vi "MEASURE_hysteresis_multiple_SHG gate_pmt.vi"() -> ()   [LabVIEW 2020]
uses:
  <vilib>/DAQmx/read.llb/DAQmx Read.vi
  <vilib>/DAQmx/read.llb/DAQmx Read (Counter U32 1Chan 1Samp).vi
  <vilib>/DAQmx/create/channels.llb/DAQmx Create Channel (CI-Count Edges).vi
  <vilib>/DAQmx/miscellaneous.llb/DAQmx Fill In Error Info.vi
  <vilib>/Utility/file.llb/Write To Spreadsheet File (DBL).vi
  <instrlib>/Stanford Research 830/Stanford Research 830.lvlib
  <instrlib>/Keithley 2450/Keithley 2450.lvlib
  <resource>/objmgr/daqmx.rc
panel:
  out "XY Graph 2":cluster{dbl[], dbl[]}(graph)
  in  "accumulation":i32=20
  in  "Interval (ms)":i32=20
  out "error out":errorcluster
  in  "Counter Channel":tag="/Dev1/PFI0"
  in  "error in":errorcluster
  out "loop run":i32
  in  "loop #":i32
  in  "Save data or not":bool=TRUE
  in  "path (folder + filename)":string="D:\\Kedar\\MoS2\\jw7_DJ_bulk_111213\\VvsHtr\\VvsHtr_300K"
  in  "Clear Plot":bool
  out "XY Graph":cluster{dbl[], dbl[]}(graph)
  out "LOCKIN Measurement":dbl
  in  "Parameter (1: X)":u16(ring)=1 items=["X"=1, "Y"=2, "R"=3, "Theta"=4, "Channel 1"=5, "Channel 2"=6, "Aux In 1"=7, "Aux In 2"=8, "Aux In 3"=9, "Aux In 4"=10]
  out "gate voltage":dbl format="%#_13g"
  out "gate leaking":string="defbuffer1"
  in  "GATE STEP(mv)":i32
  in  "GATE Low Value (default 0)":dbl=1.0
  in  "GATE High Value":dbl=1.0
  in  "Function (0: Volts) 2":u16(ring) items=["Volts", "Current", "Resistance"]
  in  "Source Compaliance":dbl=1e-06
  in  "V address":refnum<visa-resource-name>="GPIB0::24::INSTR"
  in  "SD stabilization(S) 2":dbl format="%#_13g"
  in  "Sine Output Amplitude (1 V) 2":dbl=1.0
  in  "GATE / SD stablization 3":dbl format="%#_13g"
  in  "frequency":dbl format="%#_13g"
  in  "Input Connection (0: Single-Ended Voltage)":u16(ring) items=["Single-Ended Voltage", "Differential Voltage", "1 MOhm Current Gain", "100 MOhm Current Gain"]
  in  "LOCKIN address":refnum<visa-resource-name>="GPIB0::24::INSTR"
  # "Lock-in"
  # "Gate Setting"
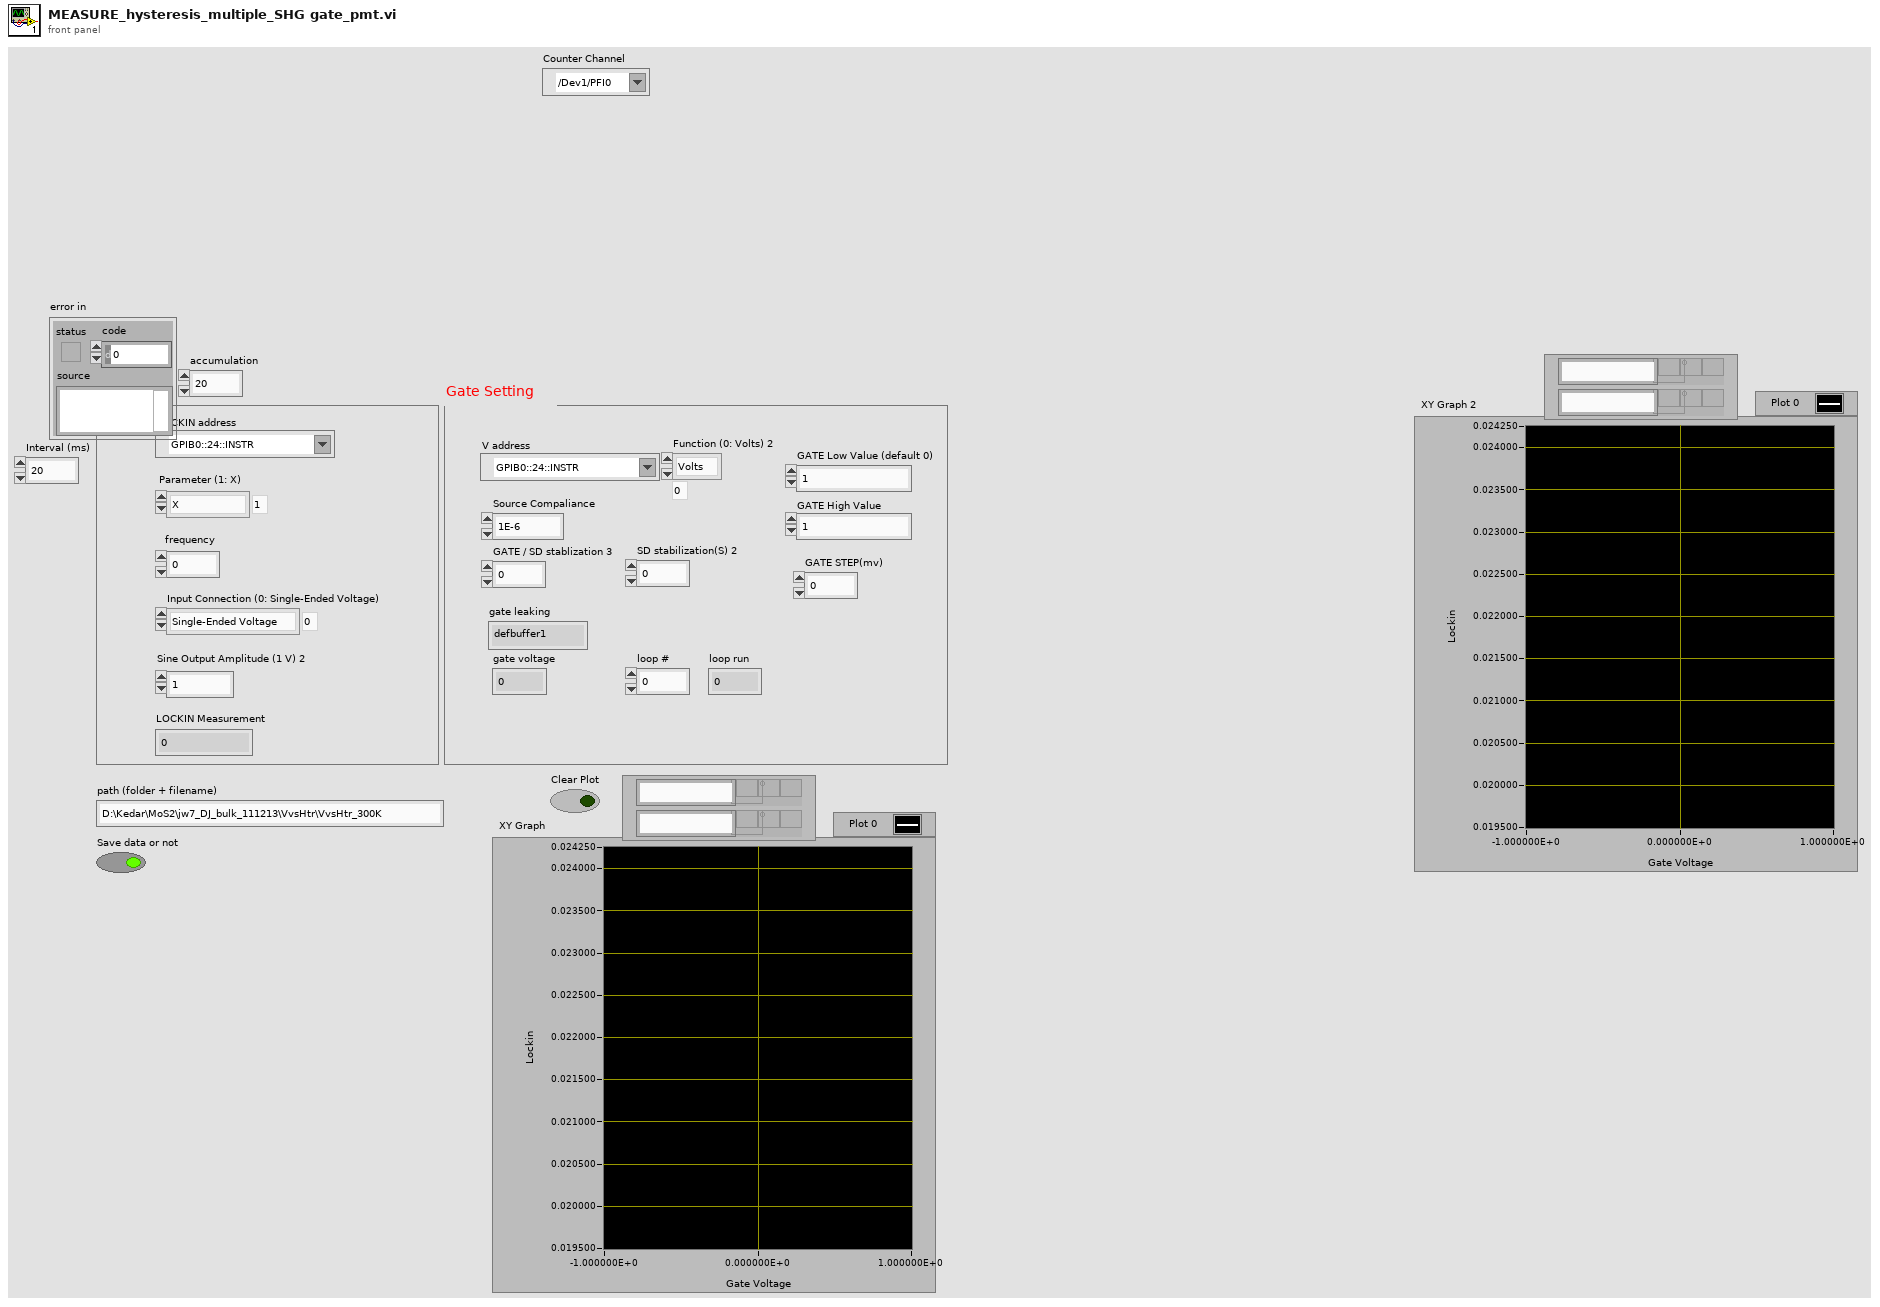
[diagram p1: front panel]
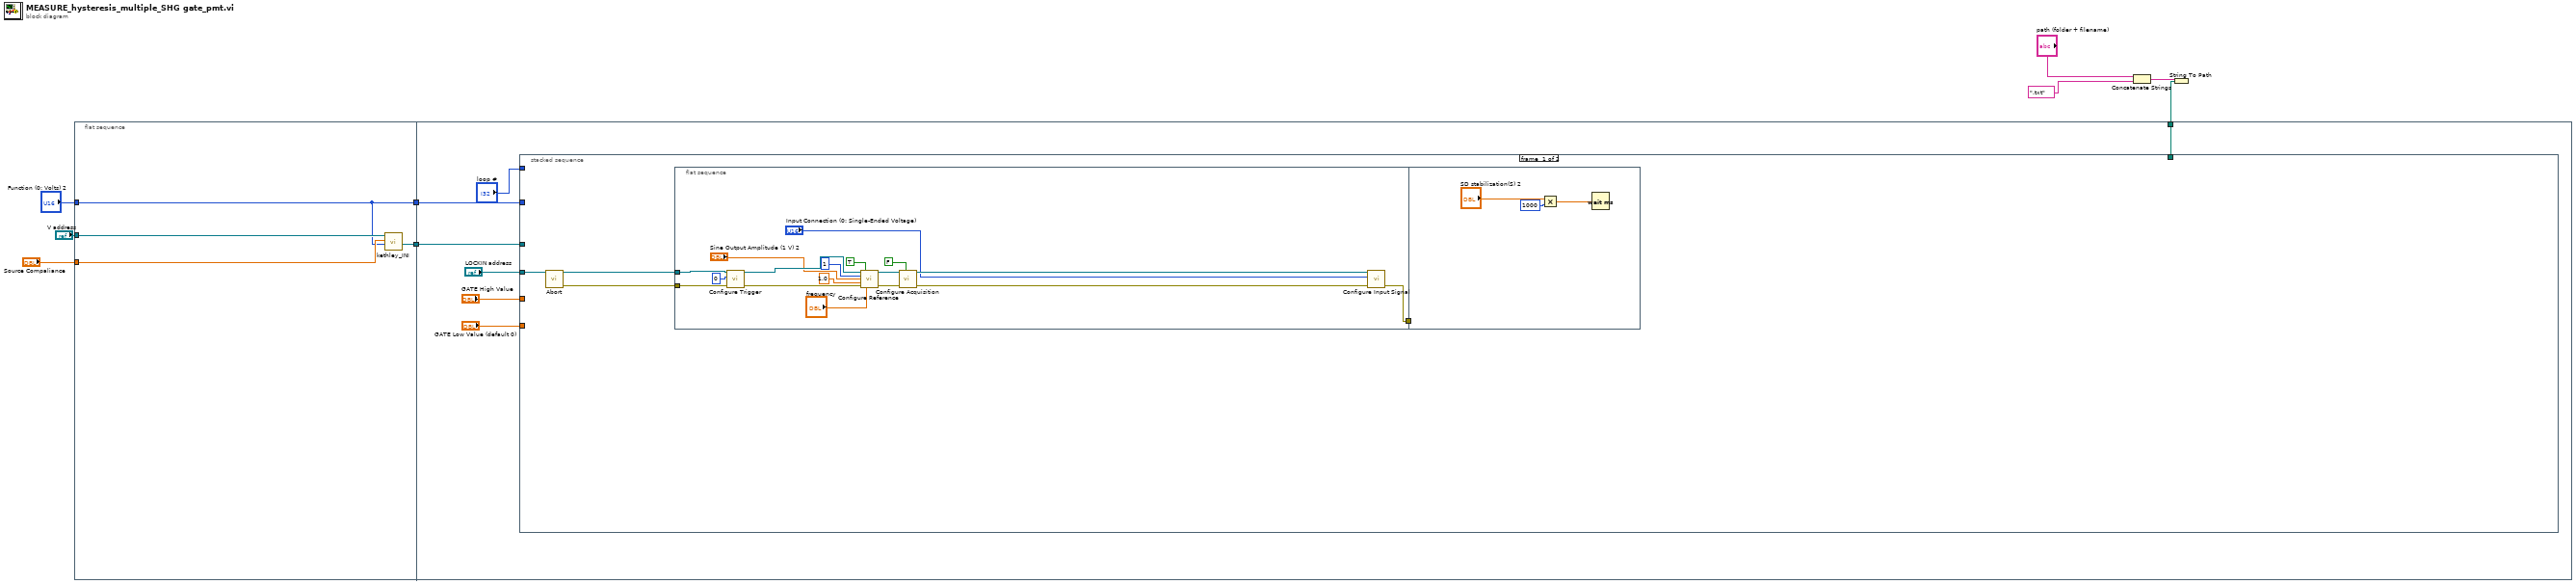
[diagram p0: block diagram]
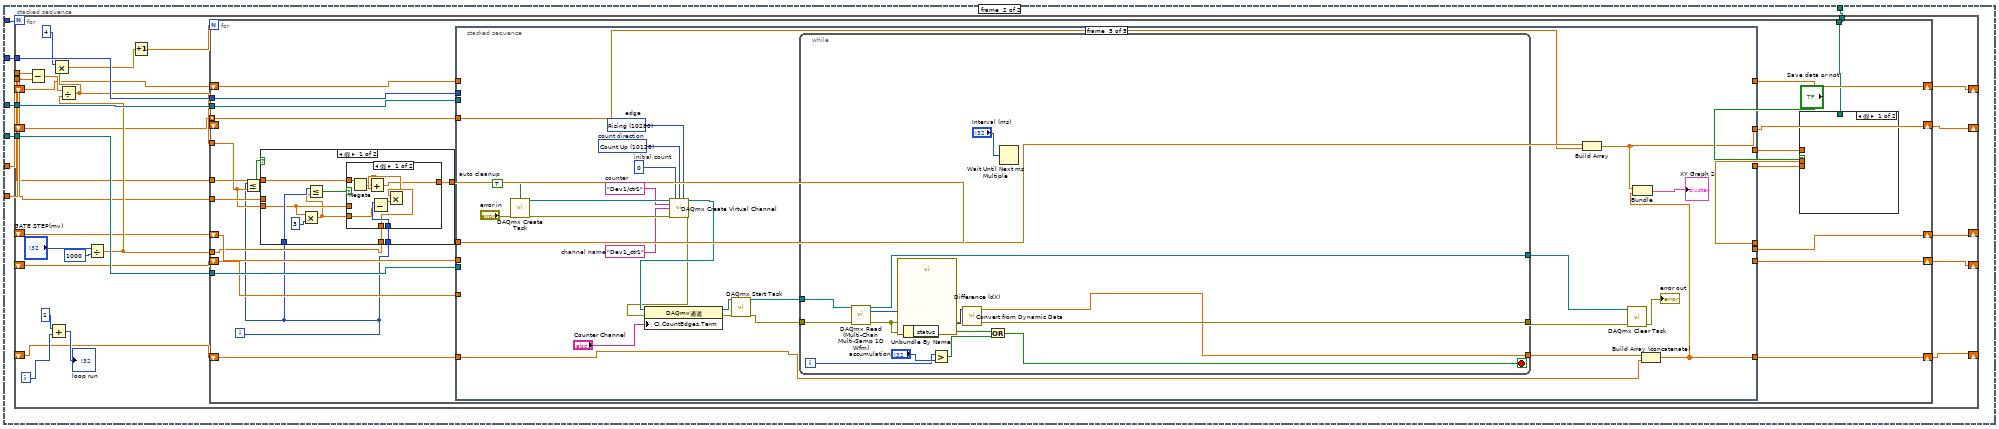
[diagram p2: hidden frame]
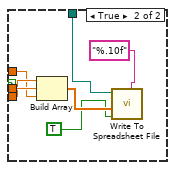
[diagram p3: hidden frame]
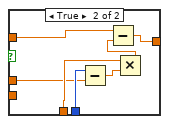
[diagram p4: hidden frame]
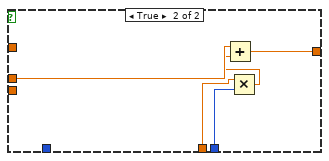
[diagram p5: hidden frame]
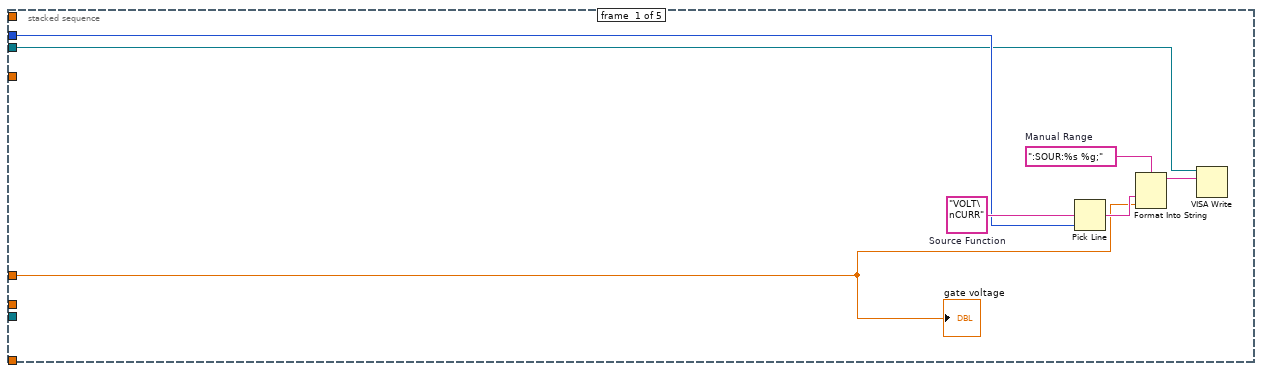
[diagram p6: hidden frame]
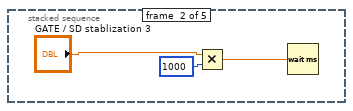
[diagram p7: hidden frame]
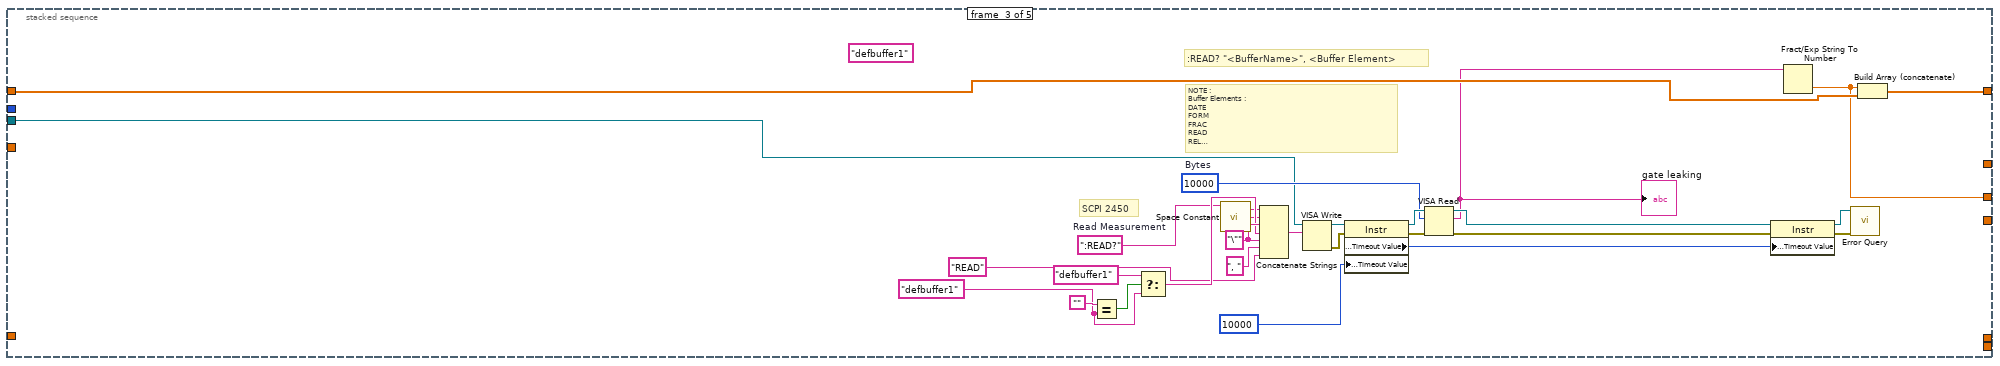
[diagram p8: hidden frame]
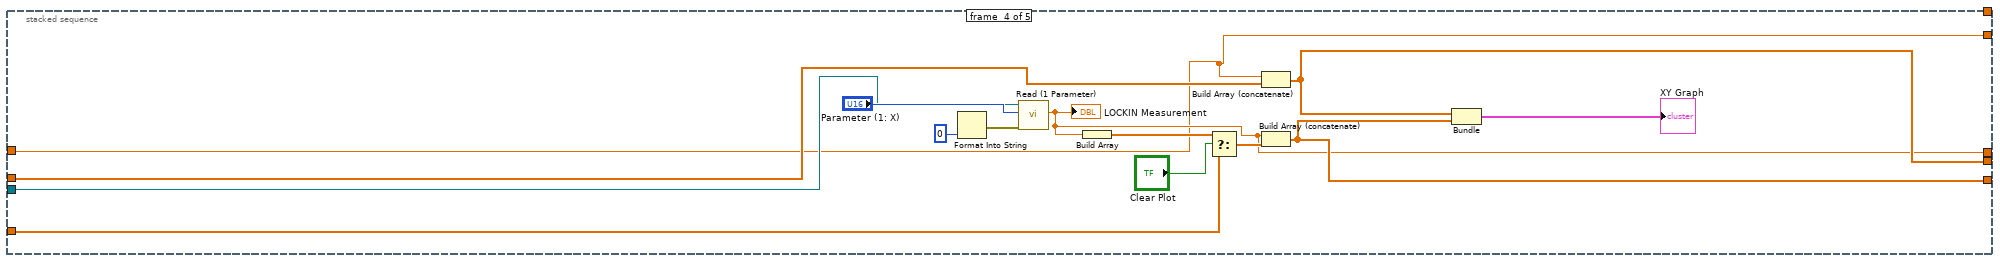
[diagram p9: hidden frame]
diagram:
  n1 = flat-sequence {
    tunnel: "V address" -> [w13]
    tunnel: "Source Compaliance" -> [w12]
    tunnel: "Function (0: Volts) 2" -> [w10]
    tunnel: [w11] -> w6
    tunnel: [w10] -> w5
    tunnel: w6 -> [w19]
    tunnel: w5 -> [w18]
    tunnel: w1 -> [w15]
    frame #0 {
      n2 = call "kethley_INI.vi"("Function (0: Volts) in"=w10, "Source Compaliance"=w12, "VISA Refnum in"=w13) -> ("VISA resource name out"=w11:refnum<visa-resource-name>)  [unwired: 8 in]
    }
    frame #1 {
      n3 = stacked-sequence {
        tunnel: "LOCKIN address" -> [w23 w49]
        tunnel: w19 -> [_ w50]
        tunnel: w18 -> [_ w51]
        tunnel: "GATE High Value" -> [_ w47]
        tunnel: "GATE Low Value (default 0)" -> [_ w48]
        tunnel: w15 -> [_ w46]
        tunnel: "loop #" -> [_ w45]
        frame #0 {
          n4 = call <instrlib>:"Abort.vi"("VISA resource name"=w23) -> ("error out"=w21:errorcluster, "VISA resource name out"=w22:refnum<visa-resource-name>)  [unwired: 9 in]
          n5 = flat-sequence {
            tunnel: w22 -> [w41]
            tunnel: [w26] -> w24
            tunnel: w21 -> [w25]
            tunnel: w24 -> [_]
            frame #0 {
              n6 = call <instrlib>:"Configure Trigger.vi"("error in (no error)"=w25, "Trigger Source (0: Internal)"=0, "VISA resource name"=w41) -> ("error out"=w35:errorcluster, "VISA resource name out"=w36:refnum<visa-resource-name>)  [unwired: 7 in]
              n7 = call <instrlib>:"Configure Reference.vi"("VISA resource name"=w36, "Auto Phase (T: Enabled)"=TRUE, "Reference Source (1: Internal)"=1, "Sine Output Amplitude (1 V)"="Sine Output Amplitude (1 V) 2", "Detection Harmonic Number (1)"=1.0 ("output voltage 2"), "error in (no error)"=w35, "Internal Reference Frequency (1000 Hz)"="frequency") -> ("VISA resource name out"=w33:refnum<visa-resource-name>, "error out"=w28:errorcluster)  [unwired: 7 in]
              n8 = call <instrlib>:"Configure Acquisition.vi"("Continuous Storage (T: Enable)"=FALSE, "error in (no error)"=w28, "VISA resource name"=w33) -> ("error out"=w27:errorcluster, "VISA resource name out"=w31:refnum<visa-resource-name>)  [unwired: 7 in]
              n9 = call <instrlib>:"Configure Input Signal.vi"("error in (no error)"=w27, "Input Connection (0: Single-Ended Voltage)"="Input Connection (0: Single-Ended Voltage)", "VISA resource name"=w31) -> ("error out"=w26:errorcluster)  [unwired: 7 in, 1 out]
            }
            frame #1 {
              n10 = Multiply(x="SD stabilization(S) 2", y=1000) -> (x*y=w44:dbl)
              n11 = Wait (ms)(milliseconds to wait=w44) -> ()  [unwired: 1 out]
            }
          }
        }
        frame #1 {
          n12 = for {
            N: w45 -> [_]
            tunnel: w51 -> [w78]
            tunnel: w50 -> [w77]
            tunnel: w49 -> [w76]
            tunnel: w48 -> [w70]
            tunnel: w47 -> [w69]
            tunnel: w46 -> [w68]
            shift-right: [w64] -> _
            shift-left: _ -> [w63]
            shift-right: [w62] -> _
            shift-left: _ -> [w60]
            shift-right: [w61] -> _
            shift-left: _ -> [w59]
            shift-right: [w55] -> _
            shift-left: _ -> [w54]
            shift-right: [w53] -> _
            shift-left: _ -> [w52]
            i -> [w57]
            n13 = Subtract(x=w69, y=w70) -> (x-y=w72:dbl)
            n14 = Add(x=1, y=w57) -> (x+y=→"loop run":i32)
            n15 = Divide(x="GATE STEP(mv)", y=1000) -> (x/y=w71:dbl)
            n16 = Divide(x=w72, y=w71) -> (x/y=w67:dbl)
            n17 = Multiply(x=4, y=w67) -> (x*y=w66:dbl)
            n18 = Increment(x=w66) -> (x+1=w65:dbl)
            n19 = for {
              N: w65 -> [_]
              tunnel: w78 -> [w103]
              tunnel: w77 -> [w102]
              tunnel: w76 -> [w101]
              tunnel: w71 -> [w92]
              shift-right: [w100] -> w64
              shift-left: w63 -> [w99]
              shift-right: [w96] -> w61
              shift-left: w59 -> [w98]
              shift-right: [w95] -> w62
              shift-left: w60 -> [w97]
              tunnel: w67 -> [w89]
              tunnel: w70 -> [w93]
              tunnel: w69 -> [w90]
              tunnel: w68 -> [w84]
              shift-right: [w82] -> w55
              shift-left: w54 -> [w81]
              shift-right: [w80] -> w53
              shift-left: _ -> [_]
              tunnel: w52 -> [w79] mode=indexing
              i -> [w88]
              n20 = Less Or Equal?(x=w88, y=w89) -> (x <= y?=w94:bool)
              n21 = case shown="假" w94 {
                tunnel: w93 -> [_ w139]
                tunnel: w88 -> [w119 w138]
                tunnel: w92 -> [w118 w137]
                tunnel: [w116 w135] -> w91
                tunnel: w90 -> [w117 _]
                tunnel: w89 -> [w112 _]
                tunnel: w88 -> [w115 _]
                frame False {
                  n22 = Multiply(x=w112, y=3) -> (x*y=w111:dbl)
                  n23 = Less Or Equal?(x=w115, y=w111) -> (x <= y?=w113:bool)
                  n24 = case shown="假" w113 {
                    tunnel: w119 -> [w127 w134]
                    tunnel: w118 -> [w125 w132]
                    tunnel: w117 -> [w121 w130]
                    tunnel: [w123 w129] -> w116
                    tunnel: w112 -> [_ w128]
                    tunnel: w111 -> [w120 _]
                    frame False {
                      n25 = Negate(x=w121) -> (-x=w122:dbl)
                      n26 = Subtract(x=w127, y=w120) -> (x-y=w126:dbl)
                      n27 = Multiply(x=w125, y=w126) -> (x*y=w124:dbl)
                      n28 = Add(x=w122, y=w124) -> (x+y=w123:dbl)
                    }
                    frame True {
                      n29 = Subtract(x=w134, y=w128) -> (x-y=w133:dbl)
                      n30 = Multiply(x=w132, y=w133) -> (x*y=w131:dbl)
                      n31 = Subtract(x=w130, y=w131) -> (x-y=w129:dbl)
                    }
                  }
                }
                frame True {
                  n32 = Multiply(x=w137, y=w138) -> (x*y=w136:dbl)
                  n33 = Add(x=w139, y=w136) -> (x+y=w135:dbl)
                }
              }
              n34 = stacked-sequence {
                tunnel: w103 -> [w142 _ _ _ _]
                tunnel: w102 -> [w141 _ w154 _ _]
                tunnel: w101 -> [_ _ _ w179 _]
                tunnel: w91 -> [w140 _ _ w177 w193]
                tunnel: [_ _ w152 _ _] -> w100
                tunnel: w99 -> [_ _ w153 _ _]
                tunnel: w98 -> [_ _ _ w183 _]
                tunnel: w97 -> [_ _ _ w180 _]
                tunnel: [_ _ _ w182 _] -> w96
                tunnel: [_ _ _ w181 _] -> w95
                tunnel: [_ _ _ w178 _] -> w87
                tunnel: [_ _ _ w177 _] -> w86
                tunnel: [_ _ w150 _ _] -> w85
                tunnel: [_ _ _ _ w194] -> w82
                tunnel: w81 -> [_ _ _ _ w196]
                tunnel: [_ _ _ _ w192] -> w80
                tunnel: w79 -> [_ _ _ _ w191]
                frame #0 {
                  w144 = "VOLT\nCURR"  # Source Function
                  w145 = ":SOUR:%s %g;"  # Manual Range
                  n35 = Pick Line(multi-line string=w144, line index=w142) -> (output string=w143:string)  [unwired: 1 out]
                  n36 = Format Into String(format string=w145, w143, w140) -> (resulting string=w146:string)  [unwired: 2 in, 1 out]
                  n37 = VISA Write(VISA resource name=w141, write buffer=w146) -> ()  [unwired: 1 in, 3 out]
                  "gate voltage" <- w140
                }
                frame #1 {
                  n38 = Multiply(x="GATE / SD stablization 3", y=1000) -> (x*y=w149:dbl)
                  n39 = Wait (ms)(milliseconds to wait=w149) -> ()  [unwired: 1 out]
                }
                frame #2 {
                  w165 = "defbuffer1" ("Buffer Name (defbuffer1) 2")
                  (unwired) "defbuffer1" ("t")
                  w163 = "\""
                  w160 = ":READ?"  # Read Measurement
                  w169 = u32 10000  # Bytes
                  # "NOTE :\nBuffer Elements :\nDATE\nFORM\nFRAC\nREAD\nREL\nSEC\nSOUR\nSOURFORM\nSOURSTAT\nSOURUNIT\nSTAT\nTIME\nTsT\nUNIT"
                  # ":READ? \"<BufferName>\", <Buffer Element>"
                  # "SCPI 2450"
                  n40 = Equal?(x="", y=w165) -> (x = y?=w166:bool)
                  n41 = Select(t="defbuffer1", s=w166, f=w165) -> (s? t:f=w162:string)
                  n42 = call <vilib>:"Space Constant.vi"() -> ("String"=w161:string)
                  n43 = Concatenate Strings(w160, w161, w163, w162, w163, ", " ("string"), "READ" ("Buffer Elements 2")) -> (w176:string)
                  n44 = VISA Write(VISA resource name=w154, write buffer=w176) -> (VISA resource name out=w168:refnum<visa-resource-name>, error out=w175:errorcluster)  [unwired: 1 in, 1 out]
                  n45 = property class="Instr"(reference=w168, error in=w175, "General Settings:Timeout Value"=10000 ("Timeout (10000 ms) 2")) -> (reference out=w174:refnum<visa-resource-name>, error out=w173:errorcluster, "General Settings:Timeout Value"=w170:u32)
                  n46 = VISA Read(VISA resource name=w174, byte count=w169, error in (no error)=w173) -> (VISA resource name out=w172:refnum<visa-resource-name>, read buffer=w151:string, error out=w171:errorcluster)  [unwired: 1 out]
                  "gate leaking" <- w151
                  n47 = property class="Instr"(reference=w172, error in=w171, "General Settings:Timeout Value"=w170) -> (reference out=w158:refnum<visa-resource-name>, error out=w157:errorcluster)
                  n48 = Fract/Exp String To Number(string=w151) -> (number=w150:dbl)  [unwired: 3 in, 1 out]
                  n49 = call <instrlib>:"Error Query.vi"("error in (no error)"=w157, "VISA resource name"=w158) -> ()  [unwired: 10 out]
                  n50 = Build Array (concatenate)(w150, w153) -> (w152:dbl[])
                }
                frame #3 {
                  n51 = Format Into String(0) -> (error out=w190:errorcluster)  [unwired: 3 in, 1 out]
                  n52 = call <instrlib>:"Read (1 Parameter).vi"("error in (no error)"=w190, "Parameter (1: X)"="Parameter (1: X)", "VISA resource name"=w179) -> ("Measurement"=w178:dbl)  [unwired: 6 in, 2 out]
                  "LOCKIN Measurement" <- w178
                  n53 = Build Array(w178) -> (w187:dbl[])
                  n54 = Select(t=w187, s="Clear Plot", f=w183) -> (s? t:f=w188:dbl[])
                  n55 = Build Array (concatenate)(w177, w180) -> (w181:dbl[])
                  n56 = Build Array (concatenate)(w178, w188) -> (w182:dbl[])
                  n57 = Bundle(w181, w182) -> (→"XY Graph":cluster{dbl[], dbl[]})  [unwired: 1 in]
                }
                frame #4 {
                  w205 = 10280 items=["Rising"=10280, "Falling"=10171]  # edge
                  w206 = 10128 items=["Count Up"=10128, "Count Down"=10124, "Externally Controlled"=10326]  # count direction
                  w207 = u32 0  # initial count
                  w208 = "Dev1_ctr1"  # channel name
                  w209 = "Dev1/ctr1"  # counter
                  w211 = TRUE  # auto cleanup
                  n58 = call <vilib>:"DAQmx Create Task.vi"("auto cleanup"=w211, "error in"="error in") -> ("task out"=w210:refnum<k21>, "error out"=w212:errorcluster)  [unwired: 12 in]
                  n59 = call-poly <vilib>:"DAQmx Create Virtual Channel.vi"("task in"=w210, "initial count"=w207, "count direction"=w206, "edge"=w205, "counter"=w209, "name to assign"=w208, "error in"=w212) -> ("task out"=w204:refnum<k21>, "error out"=w203:errorcluster)  [unwired: 7 in]
                  n60 = property class="DAQmx通道"(reference=w204, error in=w203, "CI.CountEdges.Term"="Counter Channel") -> (reference out=w216:refnum<k21>, error out=w215:errorcluster)
                  n61 = call <vilib>:"DAQmx Start Task.vi"("task/channels in"=w216, "error in"=w215) -> ("task out"=w202:refnum<k21>, "error out"=w201:errorcluster)  [unwired: 12 in]
                  n62 = while {
                    tunnel: w202 -> [w225]
                    tunnel: w201 -> [w224]
                    tunnel: [w223] -> w199
                    tunnel: [w222] -> w198
                    tunnel: [w217] -> w197
                    i -> [w219]
                    stop <- w221 stop-if-true
                    n63 = call-poly "DAQmx Read (Multi-Chan Multi-Samp 1D Wfm).vi"("task/channels in"=w225, "error in"=w224) -> ("task out"=w222:refnum<k21>, "data"=w226:u32, "error out"=w223:errorcluster)  [unwired: 11 in]
                    n64 = call "Difference (dX)"("Signals"=w226) -> ("Result"=w229:dynamicdata)  [unwired: 5 in, 1 out]
                    n65 = Unbundle By Name(w223) -> ("status"=w227:bool)
                    n66 = Greater?(x=w219, y="accumulation") -> (0:w218:bool)
                    n67 = call "Convert from Dynamic Data"("Dynamic Data Type"=w229) -> ("Scalar"=w217:dbl)  [unwired: 3 in]
                    n68 = Or(x=w227, y=w218) -> (x .or. y?=w221:bool)
                    n69 = Wait Until Next ms Multiple(millisecond multiple="Interval (ms)") -> ()  [unwired: 1 out]
                  }
                  n70 = Build Array(w193, w191) -> (w192:dbl[])
                  n71 = call <vilib>:"DAQmx Clear Task.vi"("task in"=w198, "error in"=w199) -> ("error out"=→"error out":errorcluster)  [unwired: 13 in]
                  n72 = Build Array (concatenate)(w197, w196) -> (w194:dbl[])
                  n73 = Bundle(w192, w194) -> (→"XY Graph 2":cluster{dbl[], dbl[]})  [unwired: 1 in]
                }
              }
              n74 = case shown="假" "Save data or not" {
                tunnel: w87 -> [_ w110]
                tunnel: w86 -> [_ w109]
                tunnel: w85 -> [_ w108]
                tunnel: w84 -> [_ w106]
                frame False {
                }
                frame True {
                  n75 = Build Array(w109, w110, w108) -> (w105:dbl[])
                  n76 = call-poly <vilib>:"Write To Spreadsheet File.vi"("format (%.3f)"="%.10f", "append to file? (new file:F)"=TRUE, "1D data"=w105, "file path (dialog if empty)"=w106) -> ()  [unwired: 4 in, 1 out]
                }
              }
            }
          }
        }
      }
    }
  }
  n77 = Concatenate Strings("path (folder + filename)", ".txt") -> (w2:string)
  n78 = String To Path(string=w2) -> (path=w1:path)
